vi "Median Filter.vi"(3 "Reset":bool, 4 "WindowSize":u16=10, 5 "Input":dbl) -> (2 "Output":dbl)   [LabVIEW 2017, in "ArgosLib.lvlib"]
uses:
  ArgosLib.lvlib
  <vilib>/ptbypt/NI_PtbyPt.lvlib
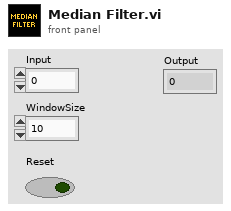
[diagram p1: front panel]
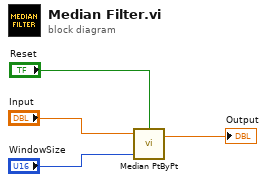
[diagram p0: block diagram]
diagram:
  n1 = call <vilib>:"Median PtByPt.vi"("initialize"="Reset", "sample length"="WindowSize", "x"="Input") -> ("median"=→"Output":dbl)  [unwired: 1 in, 1 out]
